vi "Get Plot Visibility.vi"   [LabVIEW 2019, in "Instrument UI.Lockin.lvclass"]
uses:
  Instrument UI.Lockin.lvclass
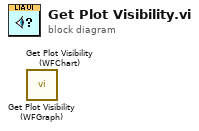
[diagram p0: block diagram]
diagram:
  n1 = call "Get Plot Visibility (WFGraph).vi"() -> ()  [unwired: 9 in, 3 out]
  n2 = call "Get Plot Visibility (WFChart).vi"() -> ()  [unwired: 9 in, 3 out]
